vi "Meas_Fast_FID_Bkgnd.vi"(3 "Mode":T5, 5 "Traverse line In":T2 {"Row Duration (mins)" format="%#.1f"; "Row No" min=0; "Trace Gas Concentration (%)" min=0.0 format="%#.2f"; "Emission Rate (l/min)" format="%#.2f"; "Tunnel Speed" format="%#.2f"; "Start X" format="%#.2f"; "Start Y" format="%#.2f"; "Start Z" format="%#.2f"; "End X" format="%#.2f"; "End Y" format="%#.2f"; "End Z" format="%#.2f"; "Averaging time (min)" min=0.0 format="%#.2f"}) -> (0 "Error Message":string, 1 "Status":T1, 2 "Traverse line Out":T2 {"Row Duration (mins)" format="%#.1f"; "Row No" min=0; "Trace Gas Concentration (%)" min=0.0 format="%#.2f"; "Emission Rate (l/min)" format="%#.2f"; "Tunnel Speed" format="%#.2f"; "Start X" format="%#.2f"; "Start Y" format="%#.2f"; "Start Z" format="%#.2f"; "End X" format="%#.2f"; "End Y" format="%#.2f"; "End Z" format="%#.2f"; "Averaging time (min)" min=0.0 format="%#.2f"})   [LabVIEW 2013]
uses:
  Gen Trav/Traverse_cluster.ctl
  Gen Trav/Spacing.ctl
  Controls/Multi_run_mode.ctl
  Controls/User_Specific_mode.ctl
  Gen Trav/Multi_Run_Status.ctl
  Gen Trav/Trav_mode.ctl
  File/Setup_Filetype.ctl
  Controls/Setup.ctl
  Controls/Save_Data.ctl
  Globals/Trav_pos_global.vi
  Globals/Preference_global.vi
panel:
  out "Initial Position":dbl[](array[numeric]) format="%#.2f"
  # "X           Y            Z"
  # "Start"
  # "End"
  # "X           Y            Z"
  # "Start"
  # "End"
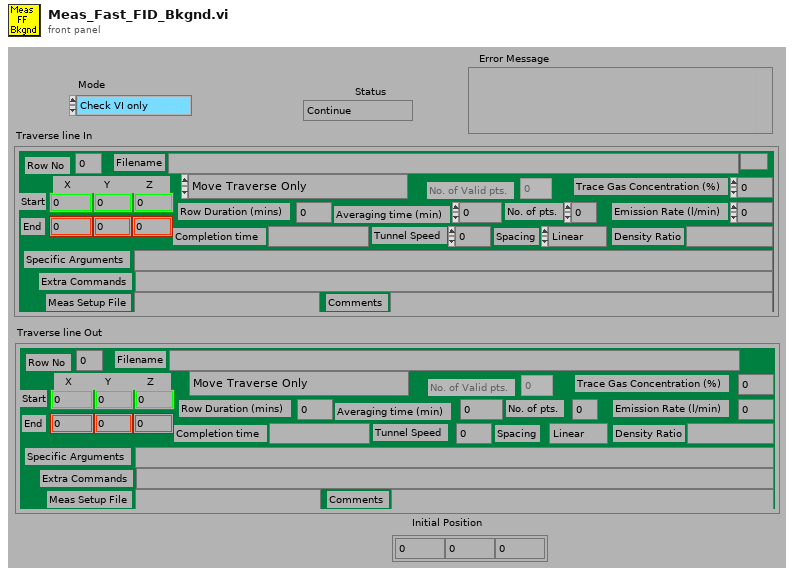
[diagram p1: front panel]
types:
  T1 = typedef "Multi_Run_Status.ctl" = enum16{"Continue", "Jump to Next Point", "Jump to Next Row", "Jump To Fall Back", "Terminate Run"}
  T2 = typedef "Traverse_cluster.ctl" = cluster{"Start X":dbl, "Start Y":dbl, "Start Z":dbl, "End X":dbl, "End Y":dbl, "End Z":dbl, "No. of pts.":i32, "Spacing":T3, "Filename":path, "Tunnel Speed":dbl, "Averaging time (min)":dbl, "Extra Commands":string, "Specific Arguments":string, "Emission Rate (l/min)":dbl, "Trace Gas Concentration (%)":dbl, "Density Ratio":string, "Comments":string, "Row No":i32, "Row Type Selector":T4, "Completion time":string, "Row Duration (mins)":dbl, "No. of Valid pts.":i32, "Meas Setup File":string}
  T3 = typedef "Spacing.ctl" = enum16{"Linear", "Log", "Gauss", "Specified", "N/A"}
  T4 = typedef "Multi_run_mode.ctl" = enum16{"Move Traverse Only", "Set Tunnel Speed Only", "Set Source Only", "Set Measurement Conditions", "Single Measurement", "Vertical Profile", "Lateral Profile", "Longitudinal Profile", "Explore Volume", "Multi-Axis Profile", "Auto Calibrate", "Meas Fast FID Bkgnd", "Check Beam Power", "Scanning Valve Measurement", "Run VI Named:", "Set ADAM Ch", "Wait (minutes)", "Send Message", "Synchronize With:", "Fall Back to this Row", "Turn Off Row Repeating", "Blank Row", "Traverse 3D Volume"}
  T5 = typedef "User_Specific_mode.ctl" = enum16{"Check VI only", "Run VI"}
  T6 = typedef "Tunnel_Coordinates.ctl" = enum16{"Work in Tunnel Coordinates", "Work in Model Coordinates"}
  T7 = typedef "Trav_mode.ctl" = enum16{"Move traverse", "Read traverse position", "Teach Position"}
  T8 = typedef "Setup_Filetype.ctl" = enum16{"Measurement Setups", "Calibration Setups", "General", "Results File Plotter Setups", "Speed Calib Tweaks"}
  T9 = typedef "Save_Data.ctl" = enum16{"Save No Data", "Save Data"}
  T10 = typedef "Setup.ctl" = enum16{"Run Program", "Show Setup", "Save Current Setup", "Setup Front Panel"}
  T11 = typedef "Status_Cluster.ctl" = cluster{"Status":T1, "Error Type":string, "Error Description":string}
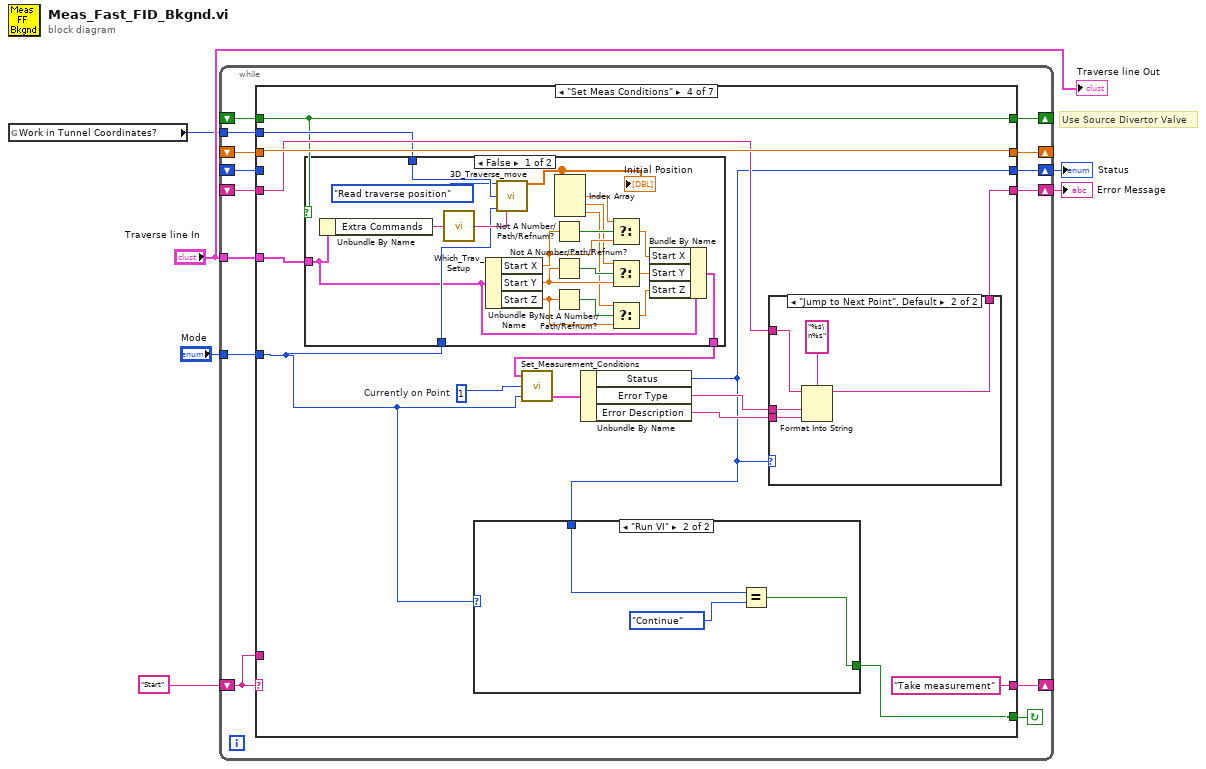
[diagram p0: block diagram]
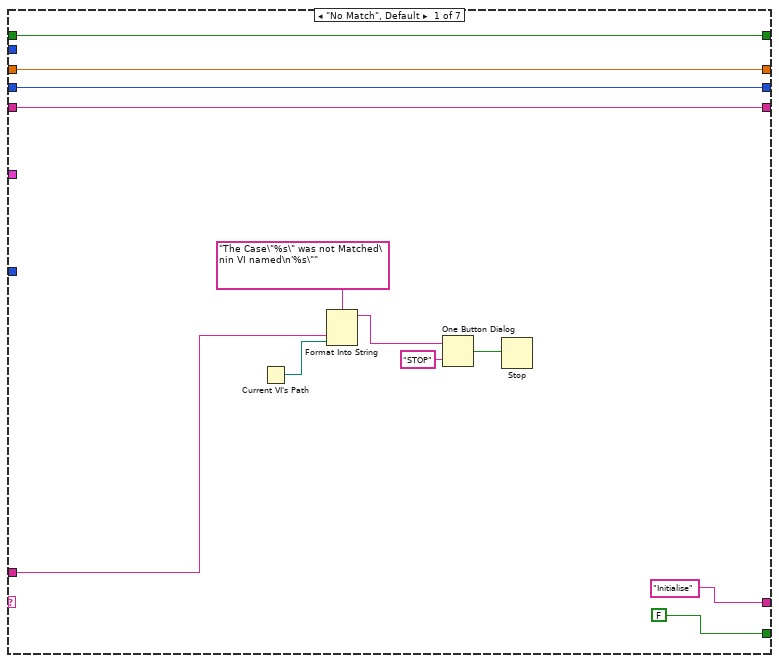
[diagram p2: hidden frame]
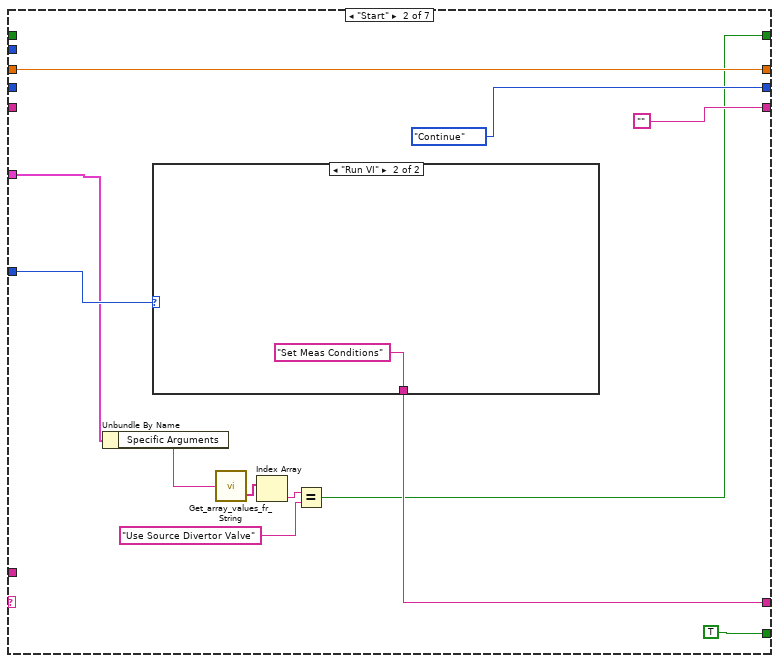
[diagram p3: hidden frame]
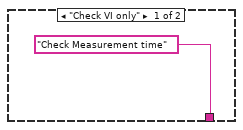
[diagram p4: hidden frame]
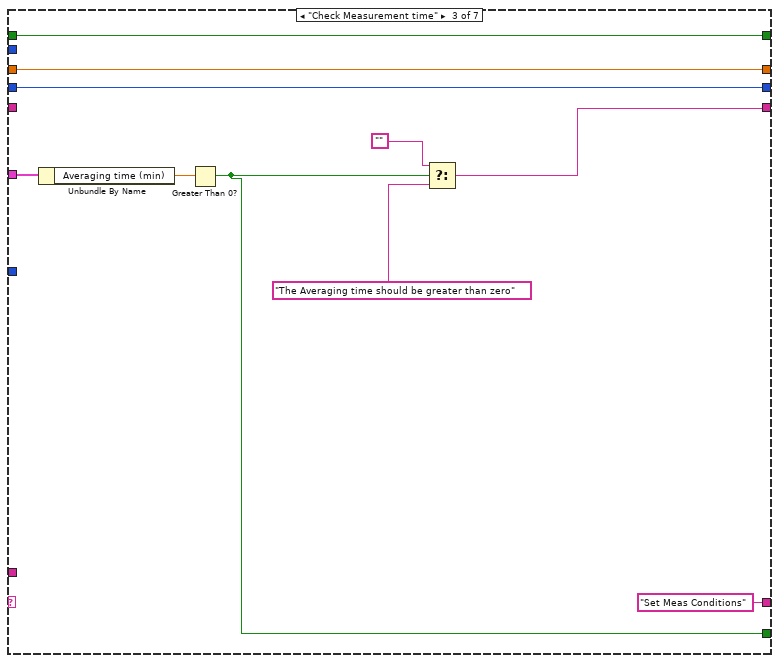
[diagram p5: hidden frame]
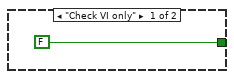
[diagram p8: hidden frame]
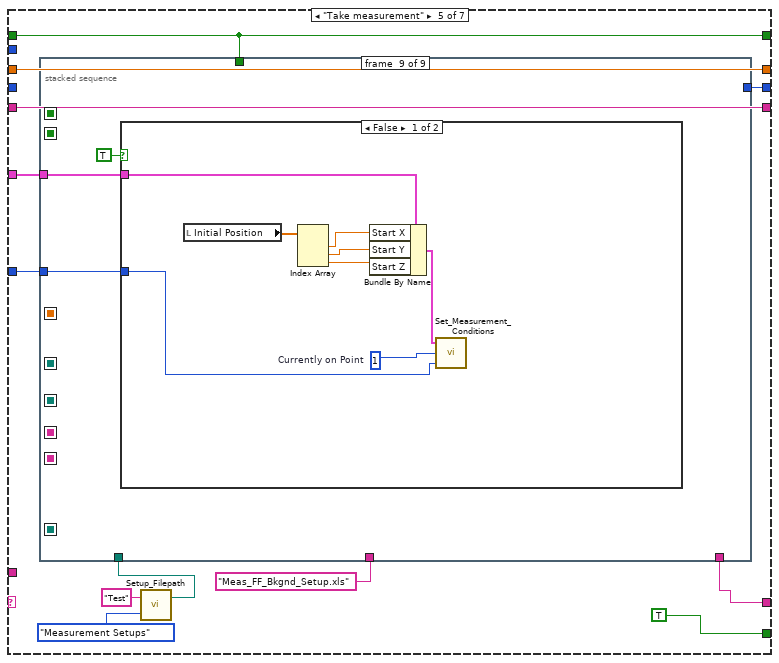
[diagram p9: hidden frame]
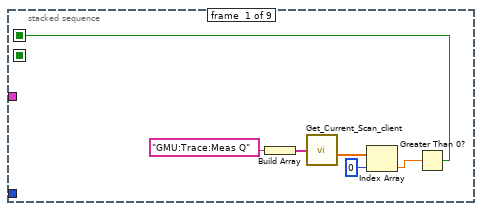
[diagram p10: hidden frame]
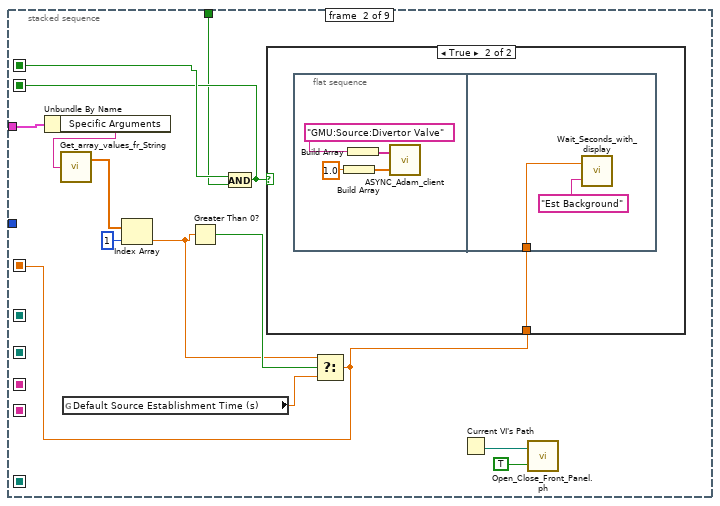
[diagram p11: hidden frame]
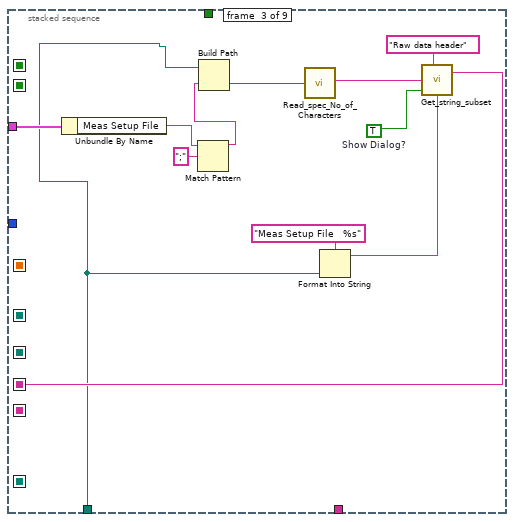
[diagram p13: hidden frame]
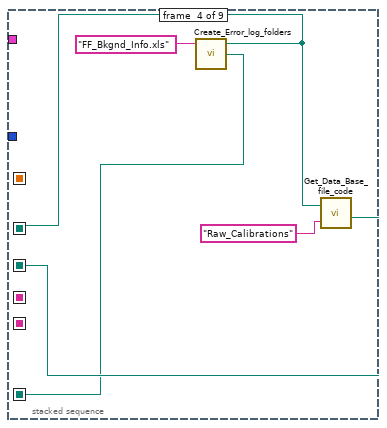
[diagram p14: hidden frame]
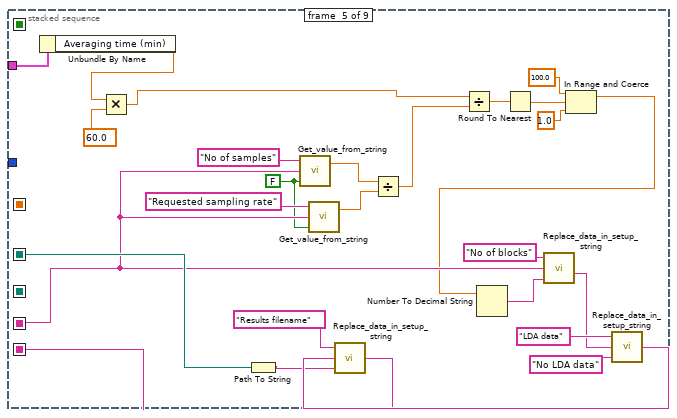
[diagram p15: hidden frame]
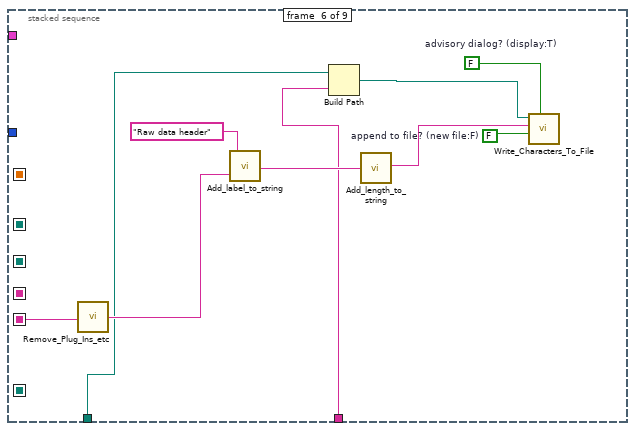
[diagram p16: hidden frame]
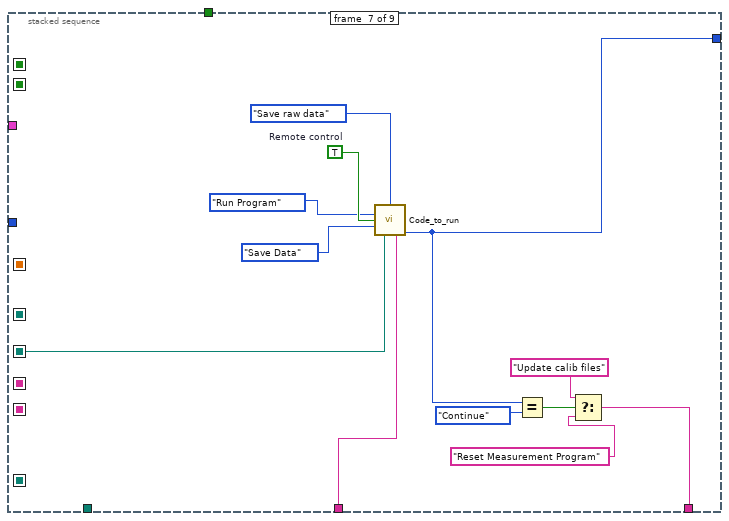
[diagram p17: hidden frame]
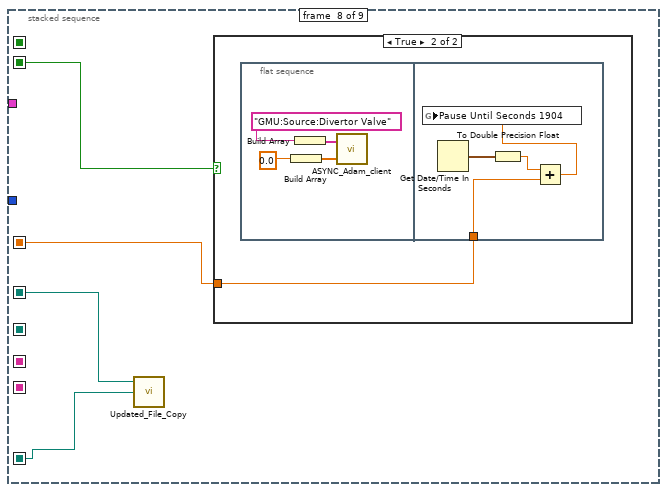
[diagram p18: hidden frame]
diagram:
  # "Use Source Divertor Valve"
  n1 = global read "Trav_pos_global.vi" "Work in Tunnel Coordinates?"() -> (w1:T6)
  n2 = while {
    shift-left: "Start" -> [w18]
    shift-right: [w19] -> _
    shift-right: [w14] -> _
    shift-left: _ -> [w17]
    tunnel: "Mode" -> [w16]
    tunnel: "Traverse line In" -> [w15]
    shift-right: [w13] -> w4
    shift-left: _ -> [w11]
    shift-right: [w12] -> w2
    shift-left: _ -> [w10]
    tunnel: w1 -> [w9]
    shift-right: [w7] -> _
    shift-left: _ -> [w8]
    stop <- w20 continue-if-true
    n3 = case shown="\"Set Meas Conditions\"" w18 {
      tunnel: [FALSE TRUE w50 w64 TRUE TRUE FALSE] -> w20
      tunnel: ["Initialise" w42 "Set Meas Conditions" "Take measurement" ("t") w108 "Reset Measurement Program" "End"] -> w19
      tunnel: w18 -> [w27 _ _ _ _ _ _]
      tunnel: w17 -> [w24 w40 w48 w69 w113 w235 _]
      tunnel: w16 -> [_ w43 _ w59 w103 _ _]
      tunnel: w15 -> [_ w36 w56 w60 w111 _ _]
      tunnel: [w24 w40 w48 w69 w113 w235 w240] -> w14
      tunnel: [w23 Multi_Run_Status."Continue" ("Status") w49 w62 w109 w234 w239] -> w13
      tunnel: [w22 "" w52 w65 w112 w233 w242] -> w12
      tunnel: w11 -> [w23 _ w49 _ _ w234 w239]
      tunnel: w10 -> [w22 _ _ w66 w112 w233 w242]
      tunnel: w9 -> [_ _ _ w58 _ _ _]
      tunnel: w8 -> [w21 _ w47 w57 w104 w230 w238]
      tunnel: [w21 w34 w47 w57 w104 w230 w238] -> w7
      frame "No Match", Default {
        n4 = Current VI's Path() -> (path=w26:path)
        n5 = Format Into String(format string="The Case\"%s\" was not Matched\nin VI named\n'%s\"" ("Format String"), w27, w26) -> (resulting string=w30:string)  [unwired: 2 in, 1 out]
        n6 = One Button Dialog(message=w30, button name ("OK")="STOP") -> (true=w28:bool)
        n7 = Stop(stop? (T)=w28) -> ()
      }
      frame "Start" {
        n8 = Unbundle By Name(w36) -> ("Specific Arguments"=w35:string)
        n9 = case shown="\"Run VI\"" w43 {
          tunnel: ["Check Measurement time" "Set Meas Conditions"] -> w42
          frame "Check VI only" {
          }
          frame "Run VI" {
          }
        }
        n10 = call "Get_array_values_fr_String.vi"("String Value"=w35) -> ("String array"=w38:string[])  [unwired: 1 out]
        n11 = Index Array(array=w38) -> (element=w37:string)  [unwired: 1 in]
        n12 = Equal?(x=w37, y="Use Source Divertor Valve") -> (x = y?=w34:bool)
      }
      frame "Check Measurement time" {
        n13 = Unbundle By Name(w56) -> ("Averaging time (min)"=w55:dbl)
        n14 = Greater Than 0?(x=w55) -> (x > 0?=w50:bool)
        n15 = Select(t="", s=w50, f="The Averaging time should be greater than zero") -> (s? t:f=w52:string)
      }
      frame "Set Meas Conditions" {
        w71 = 1  # Currently on Point
        n16 = case shown="False" w57 {
          tunnel: [w91 w92] -> w61
          tunnel: w60 -> [w73 w92]
          tunnel: w59 -> [w89 _]
          tunnel: w58 -> [w88 _]
          frame False {
            n17 = Unbundle By Name(w73) -> ("Extra Commands"=w72:string)
            n18 = call "Which_Trav_Setup.vi"("Extra Command String"=w72) -> ("Traverse Setup"=w90:string)
            n19 = Unbundle By Name(w73) -> ("Start X"=w82:dbl, "Start Y"=w78:dbl, "Start Z"=w77:dbl)
            n20 = call "3D_Traverse_move.vi"("Mode"=Trav_mode."Read traverse position", "Work in Tunnel Coordinates"=w88, "Simulate/Run"=w89, "Traverse name"=w90) -> ("Trav Position achieved"=w86:dbl[])  [unwired: 5 in, 6 out]
            "Initial Position" <- w86
            n21 = Not A Number/Path/Refnum?(number/path/refnum=w82) -> (NaN/Path/Refnum?=w85:bool)
            n22 = Not A Number/Path/Refnum?(number/path/refnum=w78) -> (NaN/Path/Refnum?=w81:bool)
            n23 = Not A Number/Path/Refnum?(number/path/refnum=w77) -> (NaN/Path/Refnum?=w80:bool)
            n24 = Index Array(array=w86) -> (element #1=w83:dbl, element #2=w76:dbl, element #3=w75:dbl)  [unwired: 3 in]
            n25 = Select(t=w83, s=w85, f=w82) -> (s? t:f=w84:dbl)
            n26 = Select(t=w76, s=w81, f=w78) -> (s? t:f=w79:dbl)
            n27 = Select(t=w75, s=w80, f=w77) -> (s? t:f=w74:dbl)
            n28 = Bundle By Name(cluster=w73, "Start X"=w84, "Start Y"=w79, "Start Z"=w74) -> (w91:T2)
          }
          frame True {
          }
        }
        n29 = call "Set_Measurement_Conditions.vi"("Simulate/Run"=w59, "Currently on Point"=w71, "Traverse line"=w61) -> ("Status Cluster"=w70:T11)  [unwired: 2 out]
        n30 = Unbundle By Name(w70) -> ("Status"=w62:T1, "Error Type"=w68:string, "Error Description"=w67:string)
        n31 = case shown="\"Run VI\"" w59 {
          tunnel: [FALSE w101] -> w64
          tunnel: w62 -> [_ w102]
          frame "Check VI only" {
          }
          frame "Run VI" {
            n32 = Equal?(x=w102, y=Multi_Run_Status."Continue" ("Status")) -> (x = y?=w101:bool)
          }
        }
        n33 = case shown="\"Jump to Next Point\", Default" w62 {
          tunnel: w68 -> [_ w98]
          tunnel: w67 -> [_ w97]
          tunnel: w66 -> [w93 w96]
          tunnel: [w93 w95] -> w65
          frame "Continue" {
          }
          frame "Jump to Next Point", Default {
            n34 = Format Into String(format string="%s\n%s", initial string=w96, w98, w97) -> (resulting string=w95:string)  [unwired: 1 in, 1 out]
          }
        }
      }
      frame "Take measurement" {
        n35 = call "Setup_Filepath.vi"("Setup File Type"=Setup_Filetype."Measurement Setups", "Filename in"="Test") -> ("Directory"=w105:path)  [unwired: 1 out]
        n36 = stacked-sequence {
          seq-local: [_ _ w150 _ _ _ _ _ _] -> [_ _ _ _ w165 _ _ _ _]
          seq-local: [_ _ _ _ w174 _ _ _ _] -> [_ _ _ _ _ w186 _ _ _]
          seq-local: [_ _ _ w154 _ _ _ _ _] -> [_ _ _ _ _ _ w201 _ _]
          seq-local: [_ _ _ w156 _ _ _ _ _] -> [_ _ _ _ w173 _ _ w209 _]
          seq-local: [_ w122 _ _ _ _ _ _ _] -> [_ _ _ _ _ _ _ w207 _]
          seq-local: [_ w124 _ _ _ _ _ _ _] -> [_ _ _ _ _ _ _ w206 _]
          seq-local: [_ _ _ w153 _ _ _ _ _] -> [_ _ _ _ _ _ _ w208 _]
          seq-local: [w115 _ _ _ _ _ _ _ _] -> [_ w123 _ _ _ _ _ _ _]
          tunnel: "Meas_FF_Bkgnd_Setup.xls" -> [_ _ _ _ _ w188 w203 _ _]
          tunnel: w111 -> [_ w131 w147 _ w169 _ _ _ w221]
          tunnel: [_ _ _ _ _ _ w199 _ _] -> w109
          tunnel: [_ _ _ _ _ _ w196 _ _] -> w108
          tunnel: w105 -> [_ _ w142 _ _ w184 _ _ _]
          tunnel: w104 -> [_ w121 _ _ _ _ _ _ _]
          tunnel: w103 -> [_ _ _ _ _ _ _ _ w220]
          frame #0 {
            n37 = Build Array("GMU:Trace:Meas Q") -> (w119:string[])
            n38 = call "Get_Current_Scan_client.vi"("ADAM Ch Names"=w119) -> ("Numerical Values"=w117:dbl[])  [unwired: 3 out]
            n39 = Index Array(array=w117, index=0) -> (element=w116:dbl)
            n40 = Greater Than 0?(x=w116) -> (x > 0?=w115:bool)
          }
          frame #1 {
            n41 = Unbundle By Name(w131) -> ("Specific Arguments"=w130:string)
            n42 = call "Get_array_values_fr_String.vi"("String Value"=w130) -> ("Numeric Array"=w128:dbl[])  [unwired: 1 out]
            n43 = global read "Preference_global.vi" "Default Source Establishment Time (s)"() -> (w125:dbl)
            n44 = Index Array(array=w128, index=1) -> (element=w126:dbl)
            n45 = Greater Than 0?(x=w126) -> (x > 0?=w127:bool)
            n46 = And(x=w123, y=w121) -> (x .and. y?=w122:bool)
            n47 = Select(t=w126, s=w127, f=w125) -> (s? t:f=w124:dbl)
            n48 = case shown="True" w122 {
              tunnel: w124 -> [_ w134]
              frame False {
              }
              frame True {
                n49 = flat-sequence {
                  tunnel: w134 -> [w139]
                  frame #0 {
                    n50 = Build Array(1.0) -> (w135:dbl[])
                    n51 = Build Array("GMU:Source:Divertor Valve") -> (w136:string[])
                    n52 = call "ASYNC_Adam_client.vi"("Values"=w135, "Channel Names"=w136) -> ()  [unwired: 2 out]
                  }
                  frame #1 {
                    n53 = call "Wait_Seconds_with_display.vi"("Message"="Est Background", "Seconds to wait"=w139) -> ()  [unwired: 2 out]
                  }
                }
              }
            }
            n54 = Current VI's Path() -> (path=w132:path)
            n55 = call "Open_Close_Front_Panel.ph.vi"("Front Panel Window:Open"=TRUE, "VI path"=w132) -> ()  [unwired: 2 out]
          }
          frame #2 {
            w148 = TRUE  # Show Dialog?
            n56 = Unbundle By Name(w147) -> ("Meas Setup File"=w145:string)
            n57 = Match Pattern(string=w145, regular expression=";") -> (before substring=w144:string)  [unwired: 4 out]
            n58 = Build Path(base path=w142, name or relative path=w144) -> (appended path=w149:path)
            n59 = call "Read_spec_No_of_Characters.vi"("Filename"=w149) -> ("character string"=w151:string)  [unwired: 1 out]
            n60 = Format Into String(format string="Meas Setup File   %s", w142) -> (resulting string=w141:string)  [unwired: 2 in, 1 out]
            n61 = call "Get_string_subset.vi"("String Name"=w141, "Show Dialog?"=w148, "String to split"=w151, "File Label"="Raw data header") -> ("Output string"=w150:string)  [unwired: 1 out]
          }
          frame #3 {
            n62 = call "Create_Error_log_folders.vi"("Log Filename"="FF_Bkgnd_Info.xls") -> ("Server copy Location"=w153:path, "Local Log File"=w156:path)  [unwired: 2 in, 1 out]
            n63 = call "Get_Data_Base_file_code.vi"("Results Filename"=w156, "Data Type"="Raw_Calibrations") -> ("Raw Data File Name"=w154:path)  [unwired: 3 out]
          }
          frame #4 {
            w162 = FALSE ("Show Dialog?")
            n64 = Unbundle By Name(w169) -> ("Averaging time (min)"=w168:dbl)
            n65 = Multiply(x=w168, y=60.0) -> (x*y=w170:dbl)
            n66 = Path To String(path=w173) -> (string=w172:string)
            n67 = call "Get_value_from_string.vi"("Show Dialog?"=w162, "Input string"=w165, "Variable name"="No of samples") -> ("Value"=w163:dbl)  [unwired: 1 out]
            n68 = call "Get_value_from_string.vi"("Show Dialog?"=w162, "Input string"=w165, "Variable name"="Requested sampling rate") -> ("Value"=w164:dbl)  [unwired: 1 out]
            n69 = Divide(x=w163, y=w164) -> (x/y=w183:dbl)
            n70 = Divide(x=w170, y=w183) -> (x/y=w182:dbl)
            n71 = Round To Nearest(number=w182) -> (nearest integer value=w161:dbl)
            n72 = In Range and Coerce(upper limit=100.0, x=w161, lower limit=1.0) -> (coerced(x)=w158:dbl)  [unwired: 1 out]
            n73 = Number To Decimal String(number=w158) -> (decimal integer string=w180:string)  [unwired: 1 out]
            n74 = call "Replace_data_in_setup_string.vi"("New data string"=w180, "Input string"=w165, "Variable name"="No of blocks") -> ("Appended string"=w177:string)
            n75 = call "Replace_data_in_setup_string.vi"("New data string"="No LDA data", "Input string"=w177, "Variable name"="LDA data" ("Label for characters")) -> ("Appended string"=w175:string)
            n76 = call "Replace_data_in_setup_string.vi"("New data string"=w172, "Input string"=w175, "Variable name"="Results filename") -> ("Appended string"=w174:string)
          }
          frame #5 {
            w192 = FALSE  # advisory dialog? (display:T)
            w193 = FALSE  # append to file? (new file:F)
            n77 = call "Remove_Plug_Ins_etc.vi"("Input String"=w186) -> ("Output string"=w185:string)
            n78 = call "Add_label_to_string.vi"("String to write"=w185, "File Label"="Raw data header") -> ("Output string"=w189:string)
            n79 = Build Path(base path=w184, name or relative path=w188) -> (appended path=w187:path)
            n80 = call "Add_length_to_string.vi"("String in"=w189) -> ("String out"=w191:string)
            n81 = call "Write_Characters_To_File.vi"("file path (dialog if empty)"=w187, "advisory dialog? (display:T)"=w192, "character string"=w191, "append to file? (new file:F)"=w193) -> ()  [unwired: 1 in, 4 out]
          }
          frame #6 {
            w205 = TRUE  # Remote control
            n82 = call "Code_to_run.vi"("Raw data option"=enum16{"Save raw data", "Raw data not saved"}."Save raw data", "setup"=Setup."Run Program", "Remote control"=w205, "File"=Save_Data."Save Data", "Raw data file"=w201, "Setup filename"=w203) -> ("Status"=w199:T1)  [unwired: 5 in, 4 out]
            n83 = Equal?(x=w199, y=Multi_Run_Status."Continue" ("Status")) -> (x = y?=w197:bool)
            n84 = Select(t="Update calib files", s=w197, f="Reset Measurement Program") -> (s? t:f=w196:string)
          }
          frame #7 {
            n85 = call "Updated_File_Copy.vi"("Target Path"=w208, "Source Path"=w209) -> ()  [unwired: 2 out]
            n86 = case shown="True" w207 {
              tunnel: w206 -> [_ w210]
              frame False {
              }
              frame True {
                n87 = flat-sequence {
                  tunnel: w210 -> [w216]
                  frame #0 {
                    n88 = Build Array(0.0) -> (w211:dbl[])
                    n89 = Build Array("GMU:Source:Divertor Valve") -> (w212:string[])
                    n90 = call "ASYNC_Adam_client.vi"("Values"=w211, "Channel Names"=w212) -> ()  [unwired: 2 out]
                  }
                  frame #1 {
                    n91 = Get Date/Time In Seconds() -> (seconds since 1Jan1904=w218:timestamp)
                    n92 = To Double Precision Float(number=w218) -> (double precision float=w217:dbl)
                    n93 = Add(x=w217, y=w216) -> (x+y=w215:dbl)
                    n94 = global write "Trav_pos_global.vi" "Pause Until Seconds 1904"(w215) -> ()
                  }
                }
              }
            }
          }
          frame #8 {
            n95 = case shown="False" TRUE {
              tunnel: w221 -> [w224 _]
              tunnel: w220 -> [w222 _]
              frame False {
                w229 = 1  # Currently on Point
                n96 = local read "Initial Position"() -> (w228:dbl[])
                n97 = Index Array(array=w228) -> (element #1=w227:dbl, element #2=w226:dbl, element #3=w225:dbl)  [unwired: 3 in]
                n98 = Bundle By Name(cluster=w224, "Start X"=w227, "Start Y"=w226, "Start Z"=w225) -> (w223:T2)
                n99 = call "Set_Measurement_Conditions.vi"("Simulate/Run"=w222, "Currently on Point"=w229, "Traverse line"=w223) -> ()  [unwired: 3 out]
              }
              frame True {
              }
            }
          }
        }
      }
      frame "Update calib files" {
        w231 = dbl[] [] ("C (ppm)")
        w232 = TRUE  # Specific Bkgnd Meas?
        n100 = call "Update_FFID_Bkgnd_info.vi"("Specific Bkgnd Meas?"=w232, "c^2 (ppm^2)"=w231, "C (ppm)"=w231) -> ()  [unwired: 1 in]
      }
      frame "Reset Measurement Program" {
        n101 = Get Date/Time In Seconds() -> (seconds since 1Jan1904=w241:timestamp)
        n102 = To Double Precision Float(number=w241) -> (double precision float=w240:dbl)
      }
    }
  }
  "Error Message" <- w2
  "Status" <- w4
  "Traverse line Out" <- "Traverse line In"
